vi "scan2d_initialize_axis.vi"(8 "error in (no error)":errorcluster, 11 "scan_2d in":refnum<class "scan_2d.lvclass">) -> (0 "error out":errorcluster, 3 "scan_2d out":refnum<class "scan_2d.lvclass">)   [LabVIEW 2015, in "scan_2d.lvclass"]
uses:
  scan_2d.lvclass
  Stage Class/Stage.lvclass
  scan_2d.lvclass/scan_2d.ctl
  UI/front_panel_class/hardware_caller_queue_numbers.ctl
  UI/panel_class/panel.lvclass
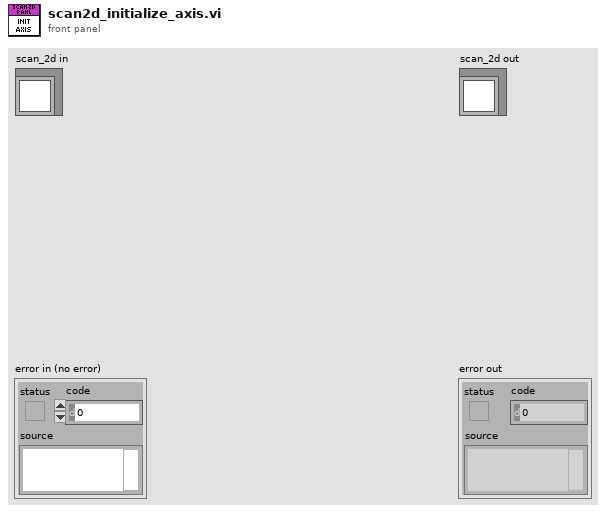
[diagram p1: front panel]
types:
  T1 = typedef "hardware_caller_queue_numbers.ctl" = enum16{"stage1", "stage2", "experiment", "detector"}
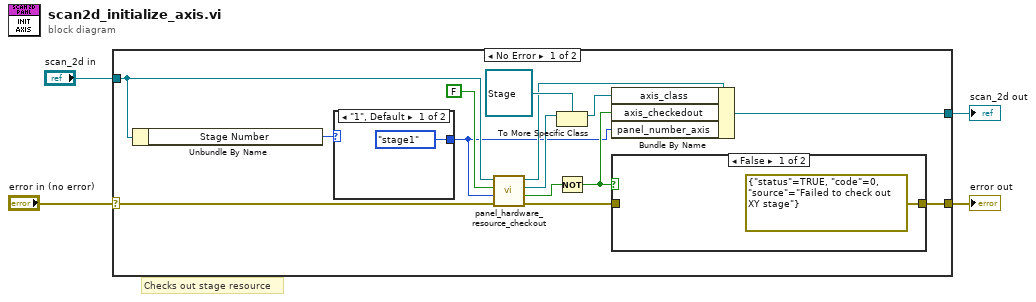
[diagram p0: block diagram]
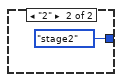
[diagram p3: hidden frame]
diagram:
  # "Checks out stage resource"
  n1 = case shown="No Error" "error in (no error)" {
    selector: "error in (no error)" -> [w15 w24]
    tunnel: [w6 w24] -> w3
    tunnel: [w9 w23] -> w1
    tunnel: "scan_2d in" -> [w16 w23]
    frame No Error {
      n2 = Unbundle By Name(w16) -> ("Stage Number"=w18:enum16{"1", "2"})
      n3 = case shown="\"1\", Default" w18 {
        tunnel: [hardware_caller_queue_numbers."stage1" ("panel_number") hardware_caller_queue_numbers."stage2" ("panel_number")] -> w5
        frame "1", Default {
        }
        frame "2" {
        }
      }
      n4 = call "panel_hardware_resource_checkout.vi"("error in (no error)"=w15, "panel_number"=w5, "Self?"=FALSE, "panel in"=w16) -> ("error out"=w8:errorcluster, "timed out?"=w10:bool, "hardware.lvclass"=w14:refnum<class "hardware.lvclass">, "panel out"=w12:refnum<class "scan_2d.lvclass">)  [unwired: 4 in]
      n5 = To More Specific Class(target class=refnum<class "Stage.lvclass"> refnum ("Stage.lvclass"), reference=w14) -> (specific class reference=w11:refnum<class "Stage.lvclass">)  [unwired: 1 in, 1 out]
      n6 = Not(x=w10) -> (.not. x?=w7:bool)
      n7 = Bundle By Name(cluster=w12, "axis_class"=w11, "axis_checkedout"=w7, "panel_number_axis"=w5) -> (w9:refnum<class "scan_2d.lvclass">)
      n8 = case shown="False" w7 {
        tunnel: w8 -> [_ w20]
        tunnel: [errorcluster {"status"=TRUE, "code"=0, "source"="Failed to check out XY stage"} ("error out") w20] -> w6
        frame False {
        }
        frame True {
        }
      }
    }
    frame Error {
    }
  }
  "error out" <- w3
  "scan_2d out" <- w1
